vi "rethinkdb_tcp_read_length.vi"(6 "timeout ms (10000)":i32=10000, 8 "error in (no error)":errorcluster, 11 "rethinkdb in":refnum<k5>) -> (0 "error out":errorcluster, 1 "response":string, 2 "token":u64 format="%016x", 3 "rethinkdb out":refnum<k5>)   [LabVIEW 2017]
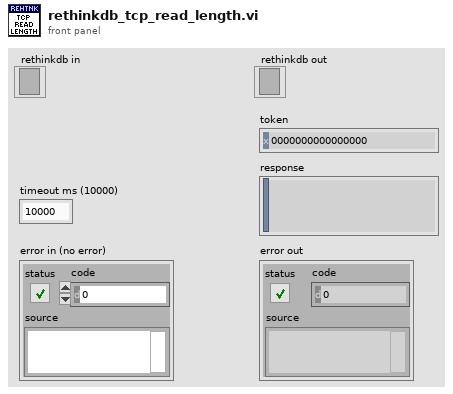
[diagram p1: front panel]
types:
  T1 = enum16{"Standard", "Buffered", "CRLF", "Immediate"}
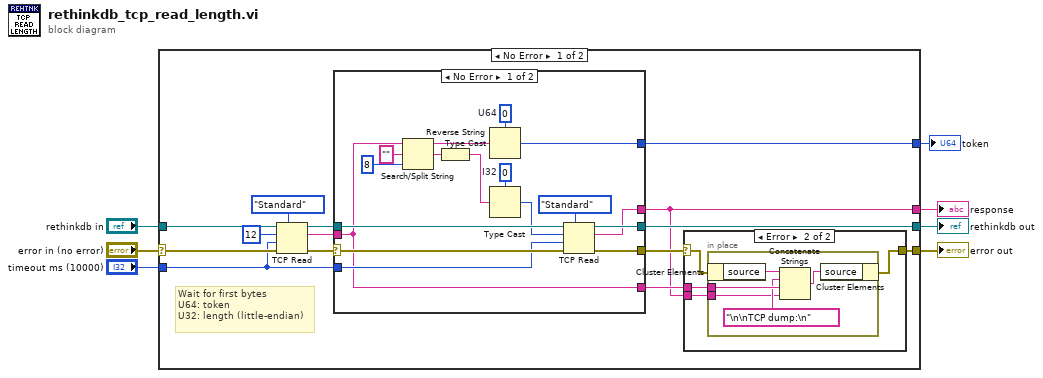
[diagram p0: block diagram]
diagram:
  n1 = case shown="No Error" "error in (no error)" {
    selector: "error in (no error)" -> [w20 w53]
    tunnel: "rethinkdb in" -> [w21 w52]
    tunnel: "timeout ms (10000)" -> [w11 _]
    tunnel: [w13 w53] -> w4
    tunnel: [w16 w52] -> w3
    tunnel: [w9 _] -> w2
    tunnel: [w8 _] -> w1
    frame No Error {
      # "Wait for first bytes\nU64: token\nU32: length (little-endian)"
      n2 = TCP Read(connection ID=w21, bytes to read=12, error in (no error)=w20, 7:T1."Standard" ("mode (standard)"), 9:w11) -> (connection ID out=w15:refnum<k5>, data out=w14:string, error out=w17:errorcluster)
      n3 = case shown="No Error" w17 {
        selector: w17 -> [w38 w41]
        tunnel: [w24 w41] -> w12
        tunnel: [w36 w40] -> w16
        tunnel: w15 -> [w37 w40]
        tunnel: w14 -> [w23 w39]
        tunnel: [w25 _] -> w9
        tunnel: w11 -> [w35 _]
        tunnel: [w23 w39] -> w10
        tunnel: [w22 _] -> w8
        frame No Error {
          w30 = 0  # I32
          w31 = u64 0  # U64
          n4 = Search/Split String(string=w23, search string/char (-)="", offset (0)=8) -> (substring before match=w32:string, match + rest of string=w29:string)  [unwired: 1 out]
          n5 = Reverse String(1:w29) -> (0:w28:string)
          n6 = Type Cast(type=w31, x=w32) -> (*(type *) &x=w22:u64)
          n7 = Type Cast(type=w30, x=w28) -> (*(type *) &x=w26:i32)
          n8 = TCP Read(connection ID=w37, bytes to read=w26, error in (no error)=w38, 7:T1."Standard" ("mode (standard)"), 9:w35) -> (connection ID out=w36:refnum<k5>, data out=w25:string, error out=w24:errorcluster)
        }
        frame Error {
        }
      }
      n9 = case shown="Error" w12 {
        selector: w12 -> [w42 w44]
        tunnel: w10 -> [_ w46]
        tunnel: [w42 w45] -> w13
        tunnel: w9 -> [_ w43]
        frame No Error {
        }
        frame Error {
          n10 = in-place {
            in-place-border: w46 -> [w49]
            in-place-border: w43 -> [w47]
            n11 = in-place-cluster #1(w44) -> ("source"=w51:string)
            n12 = Concatenate Strings(w51, "\n\nTCP dump:\n" ("format string"), w49, w47) -> (w50:string)
            n13 = in-place-cluster #1("source"=w50) -> (w45:errorcluster)
          }
        }
      }
    }
    frame Error {
    }
  }
  "error out" <- w4
  "rethinkdb out" <- w3
  "response" <- w2
  "token" <- w1
